vi "struct.vi"(8 "error in":errorcluster, 11 "struct members":T1[](array[typedef])) -> (0 "error out":errorcluster, 3 "struct string":string)   [LabVIEW 2014]
doc: "Format LV name/value pairs (both types must already be converted to strings) into an XML-RPC struct"
uses:
  structMember.ctl
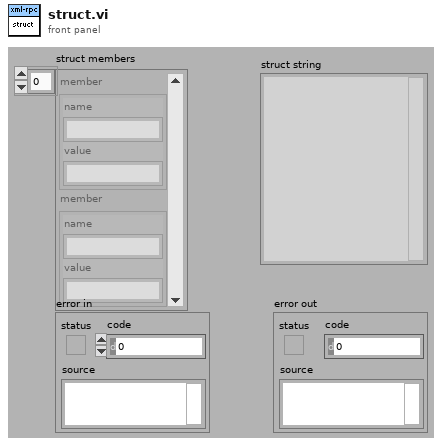
[diagram p1: front panel]
types:
  T1 = typedef "structMember.ctl" = cluster{"name":string, "value":string}
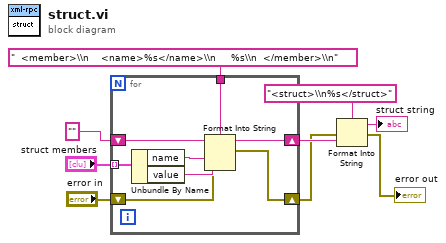
[diagram p0: block diagram]
diagram:
  n1 = for {
    tunnel: "struct members" -> [w17] mode=indexing
    shift-right: [w13] -> w4
    shift-left: "error in" -> [w14]
    tunnel: "  <member>\\n    <name>%s</name>\\n     %s\\n  </member>\\n" ("format string") -> [w12]
    shift-right: [w11] -> w5
    shift-left: "" -> [w10]
    n2 = Unbundle By Name(w17) -> ("name"=w16:string, "value"=w15:string)
    n3 = Format Into String(format string=w12, initial string=w10, error in=w14, w16, w15) -> (resulting string=w11:string, error out=w13:errorcluster)
  }
  n4 = Format Into String(format string="<struct>\\n%s</struct>", error in=w4, w5) -> (resulting string=→"struct string":string, error out=→"error out":errorcluster)  [unwired: 1 in]
